vi "Deep Copy Priv.vi"(0 "Tree Dictionary In":variant, 2 "New Parent ID":string, 7 "Unique ID":string, 11 "error in":errorcluster) -> (4 "Tree Dictionary Out":variant, 8 "ID":string, 15 "error out":errorcluster)   [LabVIEW 2020, in "NI_VIAnCFGDataStructure.lvlib" / "Tree.lvclass"]
uses:
  <vilib>/addons/analyzer/VIAnCFGDataStructure/Tree Manager/Tree.lvclass
  <vilib>/addons/analyzer/VIAnCFGDataStructure/Tree Manager/Typedefs/Tree Cluster.ctl
  <vilib>/addons/analyzer/VIAnCFGDataStructure/Tree Data/Tree Data.lvclass
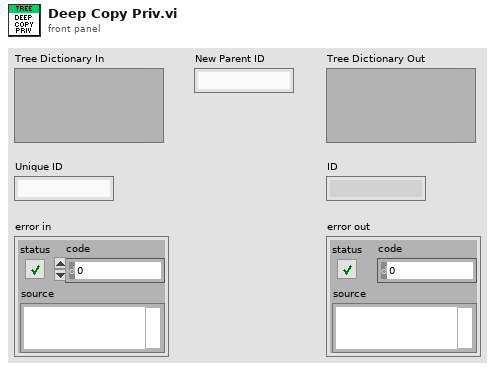
[diagram p1: front panel]
types:
  T1 = typedef "NI_VIAnCFGDataStructure.lvlib/Tree.lvclass/Tree Cluster.ctl" = cluster{"Unique ID":string, "Parent ID":string, "Child IDs":string[], "Name":string, "MetaData":string, "Data IDs":string[]}
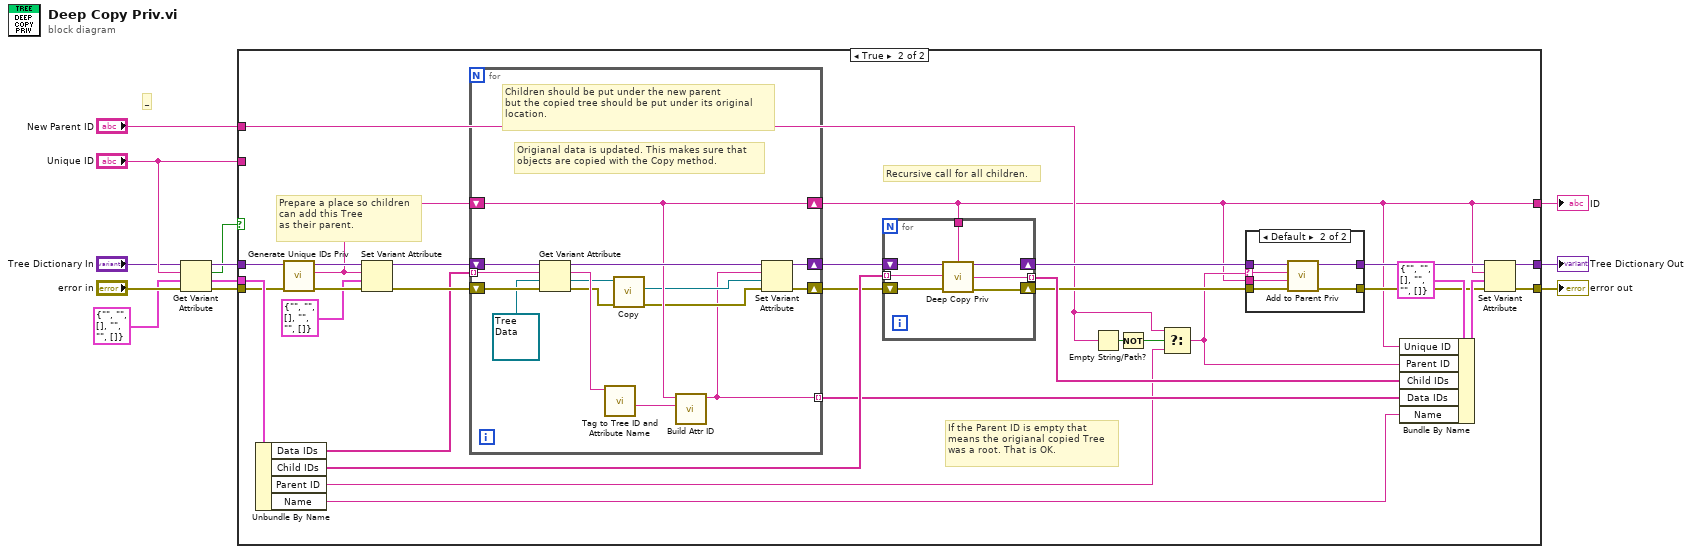
[diagram p0: block diagram]
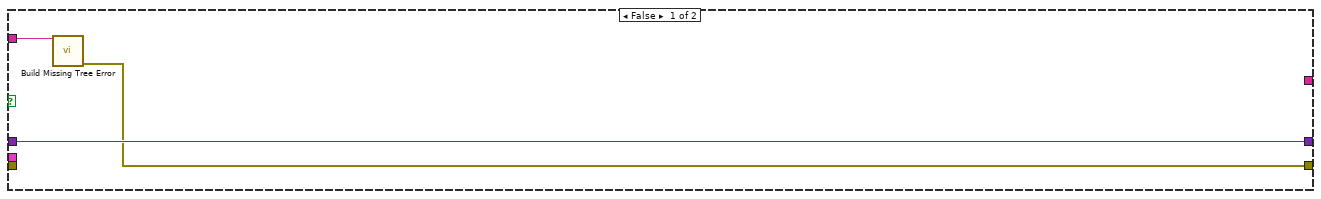
[diagram p2: hidden frame]
diagram:
  # "_"
  n1 = Get Variant Attribute(Variant="Tree Dictionary In", name="Unique ID", default value (empty Variant)=T1 {"Unique ID"="", "Parent ID"="", "Child IDs"=[], "Name"="", "MetaData"="", "Data IDs"=[]} ("Cluster of class private data"), error in="error in") -> (duplicate Variant=w6:variant, found=w4:bool, value=w5:T1, error out=w7:errorcluster)
  n2 = case shown="True" w4 {
    tunnel: w5 -> [_ w45]
    tunnel: w6 -> [w15 w39]
    tunnel: w7 -> [_ w38]
    tunnel: [w13 w27] -> w10
    tunnel: [w15 w28] -> w9
    tunnel: "Unique ID" -> [w14 _]
    tunnel: [_ w18] -> w3
    tunnel: "New Parent ID" -> [_ w35]
    frame False {
      n3 = call <vilib>:"Build Missing Tree Error.vi"("Unique ID"=w14) -> ("Error Out"=w13:errorcluster)  [unwired: 14 in]
    }
    frame True {
      # "Prepare a place so children\ncan add this Tree\nas their parent."
      # "If the Parent ID is empty that\nmeans the origianal copied Tree\nwas a root. That is OK."
      # "Recursive call for all children."
      n4 = Unbundle By Name(w45) -> ("Data IDs"=w20:string[], "Child IDs"=w43:string[], "Parent ID"=w19:string, "Name"=w17:string)
      n5 = call <vilib>:"Generate Unique IDs Priv.vi"("Error In"=w38, "Tree Dictionary"=w39) -> ("Error Out"=w33:errorcluster, "First ID"=w22:string, "Tree Dictionary Out"=w34:variant)  [unwired: 6 in, 1 out]
      n6 = Set Variant Attribute(Variant=w34, name=w22, value=T1 {"Unique ID"="", "Parent ID"="", "Child IDs"=[], "Name"="", "MetaData"="", "Data IDs"=[]} ("output cluster"), error in=w33) -> (Variant out=w25:variant, error out=w23:errorcluster)  [unwired: 1 out]
      n7 = for {
        shift-right: [w52] -> w24
        shift-left: w23 -> [w58]
        shift-right: [w53] -> w26
        shift-left: w25 -> [w59]
        tunnel: w20 -> [w56] mode=indexing
        shift-right: [w49] -> w18
        shift-left: w22 -> [w49]
        tunnel: [w46] -> w21 mode=indexing
        # "Children should be put under the new parent\nbut the copied tree should be put under its original\nlocation."
        # "Origianal data is updated. This makes sure that\nobjects are copied with the Copy method."
        n8 = Get Variant Attribute(Variant=w59, name=w56, default value (empty Variant)=refnum<class "Tree Data.lvclass"> refnum ("Tree API.lvlib:Tree Data.lvclass"), error in=w58) -> (duplicate Variant=w54:variant, value=w55:refnum<class "Tree Data.lvclass">, error out=w51:errorcluster)  [unwired: 1 out]
        n9 = call <vilib>:"Tag to Tree ID and Attribute Name.vi"("Tag"=w56) -> ("Attribute Name"=w50:string)  [unwired: 8 in, 2 out]
        n10 = call-dynamic "Copy.vi"("Error In"=w51, "Tree Data"=w55) -> ("Error Out"=w47:errorcluster, "Copy"=w48:refnum<class "Tree Data.lvclass">)  [unwired: 8 in]
        n11 = call <vilib>:"Build Attr ID.vi"("Attr Name"=w50, "Unique ID"=w49) -> ("Attr ID Out"=w46:string)  [unwired: 9 in]
        n12 = Set Variant Attribute(Variant=w54, name=w46, value=w48, error in=w47) -> (Variant out=w53:variant, error out=w52:errorcluster)  [unwired: 1 out]
      }
      n13 = for {
        shift-right: [w65] -> w40
        shift-left: w26 -> [w66]
        shift-right: [w63] -> w41
        shift-left: w24 -> [w64]
        tunnel: w43 -> [w62] mode=indexing
        tunnel: [w61] -> w42 mode=indexing
        tunnel: w18 -> [w60]
        n14 = call <vilib>:"Deep Copy Priv.vi"("Tree Dictionary In"=w66, "New Parent ID"=w60, "Unique ID"=w62, "error in"=w64) -> ("Tree Dictionary Out"=w65:variant, "ID"=w61:string, "error out"=w63:errorcluster)  [unwired: 9 in]
      }
      n15 = Empty String/Path?(string/path=w35) -> (empty?=w37:bool)
      n16 = Not(x=w37) -> (.not. x?=w36:bool)
      n17 = Select(t=w35, s=w36, f=w19) -> (s? t:f=w31:string)
      n18 = case shown="Default" w31 {
        selector: w31 -> [_ w69]
        tunnel: w40 -> [w68 w74]
        tunnel: w41 -> [w67 w73]
        tunnel: [w67 w72] -> w29
        tunnel: [w68 w71] -> w30
        tunnel: w18 -> [_ w70]
        frame "" {
        }
        frame Default {
          n19 = call <vilib>:"Add to Parent Priv.vi"("Error In"=w73, "Unique ID"=w70, "Parent ID"=w69, "Tree Dictionary"=w74) -> ("Error Out"=w72:errorcluster, "Tree Dictionary Out"=w71:variant)  [unwired: 6 in]
        }
      }
      n20 = Bundle By Name(cluster=T1 {"Unique ID"="", "Parent ID"="", "Child IDs"=[], "Name"="", "MetaData"="", "Data IDs"=[]} ("output cluster"), "Unique ID"=w18, "Parent ID"=w31, "Child IDs"=w42, "Data IDs"=w21, "Name"=w17) -> (w44:T1)
      n21 = Set Variant Attribute(Variant=w30, name=w18, value=w44, error in=w29) -> (Variant out=w28:variant, error out=w27:errorcluster)  [unwired: 1 out]
    }
  }
  "error out" <- w10
  "Tree Dictionary Out" <- w9
  "ID" <- w3
